vi "Configure Multi Eval Meas Limit ACLR UTRA Channel Bandwidth.vi"(0 "VISA resource name":refnum<visa-resource-name>, 1 "Relative Level Enabled (Value)":i32(ring)=2 items=["Off", "On", "Value"], 2 "Absolute Level Enabled (Off)":i32(ring) items=["Off", "On", "Value"], 5 "Instance (1)":T3=1, 7 "UTRA (First adjacent)":T2=1 items=["First adjacent"=1, "Second adjacent"=2], 9 "Bandwidth (5 MHz)":T1=5 items=["5 MHz"=5, "10 MHz"=10, "15 MHz"=15, "20 MHz"=20, "25 MHz"=25, "30 MHz"=30, "40 MHz"=40, "50 MHz"=50, "60 MHz"=60, "80 MHz"=80, "90 MHz"=90, "100 MHz"=100], 11 "error in (no error)":errorcluster, 12 "Relative Level (0.0)":dbl format="%^.3e", 13 "Absolute Level (0.0)":dbl format="%^.3e") -> (4 "VISA resource name out":refnum<visa-resource-name>, 15 "error out":errorcluster)   [LabVIEW 2020, in "Rohde&Schwarz CMWXP NR FR1 Measurement.lvlib"]
doc: "Defines relative and absolute limits for the ACLR measured in the first or second adjacent UTRA channel, depending on UTRA<no> (for NR SA). The settings are defined separately for each channel bandwidth.\n\nAttribute:\nRSCMWXPNRFR1M_ATTR_MULTI_EVAL_MEAS_LIMIT_ACLR_UTRA_CHANNEL_BANDWIDTH\n\nRemote-control command:\nCONFigure:NRSub:MEAS<i>:MEValuation:LIMit:ACLR:UTRA<no>:CBANdwidth<bw>"
uses:
  <instrlib>/Rohde&Schwarz CMWXP NR FR1 Measurement/Rohde&Schwarz CMWXP NR FR1 Measurement.lvlib
  <instrlib>/Rohde&Schwarz CMWXP NR FR1 Measurement/Private/_Instance.ctl
  <instrlib>/Rohde&Schwarz CMWXP NR FR1 Measurement/Private/_UTRA.ctl
  <instrlib>/Rohde&Schwarz CMWXP NR FR1 Measurement/Private/_Bandwidth.ctl
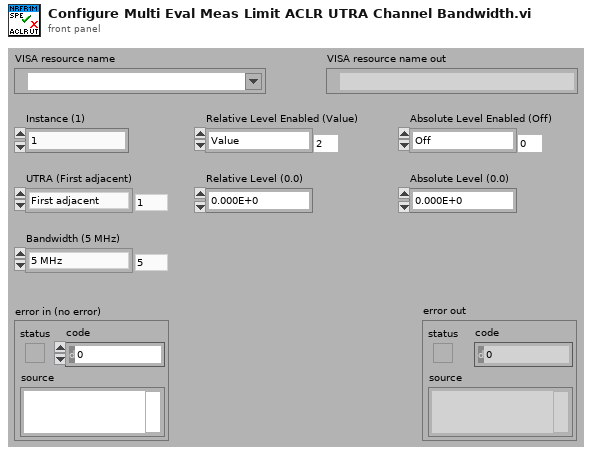
[diagram p1: front panel]
types:
  T1 = typedef "Rohde&Schwarz CMWXP NR FR1 Measurement.lvlib/_Bandwidth.ctl" = i32
  T2 = typedef "Rohde&Schwarz CMWXP NR FR1 Measurement.lvlib/_UTRA.ctl" = i32
  T3 = typedef "Rohde&Schwarz CMWXP NR FR1 Measurement.lvlib/_Instance.ctl" = i32
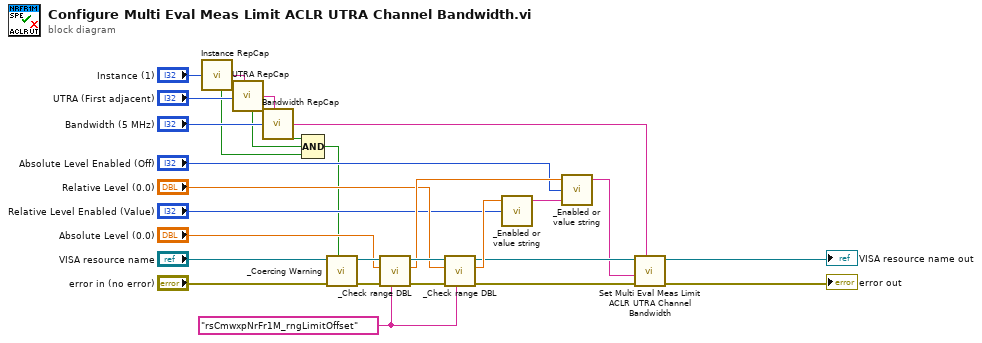
[diagram p0: block diagram]
diagram:
  w25 = "rsCmwxpNrFr1M_rngLimitOffset" ("Range Table Identifier")
  n1 = call <instrlib>:"Instance RepCap.vi"("Instance In"="Instance (1)") -> ("In Range?"=w4:bool, "RepCap Identifier Out"=w14:string)  [unwired: 1 in]
  n2 = call <instrlib>:"UTRA RepCap.vi"("UTRA In"="UTRA (First adjacent)", "RepCap String In (\"\")"=w14) -> ("In Range?"=w3:bool, "RepCap Identifier Out"=w8:string)
  n3 = call <instrlib>:"Bandwidth RepCap.vi"("Bandwidth (5 MHz)"="Bandwidth (5 MHz)", "RepCap String In (\"\")"=w8) -> ("In Range?"=w2:bool, "RepCap Identifier Out"=w7:string)
  n4 = Compound Arithmetic op=AND(w2, w3, w4) -> (w1:bool)
  n5 = call <instrlib>:"_Coercing Warning.vi"("In Range?"=w1, "error in (no error)"="error in (no error)", "VISA resource name"="VISA resource name") -> ("error out"=w29:errorcluster, "VISA resource name out"=w28:refnum<visa-resource-name>)  [unwired: 7 in]
  n6 = call <instrlib>:"_Check range DBL.vi"("Range Table Identifier"=w25, "error in (no error)"=w29, "DBL Value In"="Absolute Level (0.0)", "VISA resource name"=w28) -> ("error out"=w27:errorcluster, "DBL Value Out"=w23:dbl, "VISA resource name out"=w26:refnum<visa-resource-name>)  [unwired: 5 in]
  n7 = call <instrlib>:"_Check range DBL.vi"("Range Table Identifier"=w25, "error in (no error)"=w27, "DBL Value In"="Relative Level (0.0)", "VISA resource name"=w26) -> ("error out"=w22:errorcluster, "DBL Value Out"=w24:dbl, "VISA resource name out"=w21:refnum<visa-resource-name>)  [unwired: 5 in]
  n8 = call <instrlib>:"_Enabled or value string.vi"("Enabled or Value"="Relative Level Enabled (Value)", "Value"=w24) -> ("Resulting String"=w5:string)  [unwired: 3 in]
  n9 = call <instrlib>:"_Enabled or value string.vi"("Initial String"=w5, "Enabled or Value"="Absolute Level Enabled (Off)", "Value"=w23) -> ("Resulting String"=w6:string)  [unwired: 2 in]
  n10 = call "Set Multi Eval Meas Limit ACLR UTRA Channel Bandwidth"("Repeated Capabilities"=w7, "error in (no error)"=w22, "Multi Eval Meas Limit ACLR UTRA Channel Bandwidth ()"=w6, "instrument handle"=w21) -> ("error out"=→"error out":errorcluster, "instrument handle out"=→"VISA resource name out":refnum<visa-resource-name>)  [unwired: 6 in]
